vi "ex4.vi"() -> ()   [LabVIEW 2022 SP3]
panel:
  in  "OK Button":bool
  in  "stop":bool
  in  "username":string
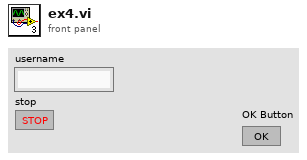
[diagram p1: front panel]
types:
  T1 = enum16{"open", "replace", "create", "open or create", "replace or create", "replace or create with confirmation"}
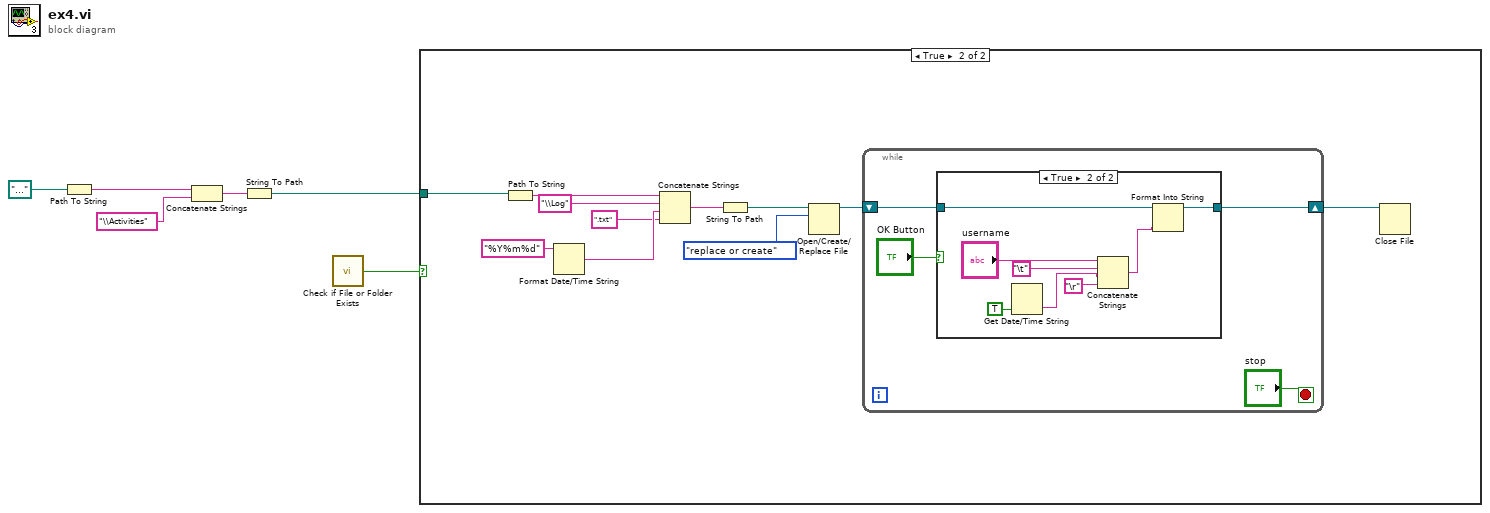
[diagram p0: block diagram]
diagram:
  n1 = Path To String(path=path "..." ("file (use dialog)")) -> (string=w5:string)
  n2 = Concatenate Strings(w5, "\\Activities" ("string")) -> (w3:string)
  n3 = String To Path(string=w3) -> (path=w1:path)
  n4 = call <vilib>:"Check if File or Folder Exists.vi"() -> ("file or folder exists?"=w2:bool)  [unwired: 9 in, 2 out]
  n5 = case shown="True" w2 {
    tunnel: w1 -> [_ w17]
    frame False {
    }
    frame True {
      n6 = Path To String(path=w17) -> (string=w16:string)
      n7 = Format Date/Time String(time format string (%c)="%Y%m%d") -> (date/time string=w14:string)  [unwired: 2 in]
      n8 = Concatenate Strings(w16, "\\Log" ("string"), w14, ".txt" ("string")) -> (w11:string)
      n9 = String To Path(string=w11) -> (path=w10:path)
      n10 = Open/Create/Replace File(file path (use dialog)=w10, operation (0:open)=T1."replace or create") -> (refnum out=w8:refnum<file>)  [unwired: 4 in, 2 out]
      n11 = while {
        shift-right: [w20] -> w7
        shift-left: w8 -> [w21]
        stop <- "stop" stop-if-true
        n12 = case shown="True" "OK Button" {
          tunnel: w21 -> [w22 w25]
          tunnel: [w22 w23] -> w20
          frame False {
          }
          frame True {
            n13 = Get Date/Time String(want seconds? (F)=TRUE) -> (time string=w27:string)  [unwired: 2 in, 1 out]
            n14 = Concatenate Strings("username", "\t", w27, "\r") -> (w24:string)
            n15 = Format Into String(initial string=w25, w24) -> (resulting string=w23:refnum<file>)  [unwired: 2 in, 1 out]
          }
        }
      }
      n16 = Close File(refnum=w7) -> ()  [unwired: 1 in, 2 out]
    }
  }
